vi "Get Node.vi"(8 "error in (no error)":errorcluster, 10 "Path in":string, 11 "Connection in":refnum<class "Connection.lvclass">) -> (0 "error out":errorcluster, 2 "Node out":refnum<class "TreeNode.lvclass">, 3 "Connection out":refnum<class "Connection.lvclass">)   [LabVIEW 2015, in "MDSplus.lvlib" / "Connection.lvclass"]
uses:
  <vilib>/MDSplus_LV2015/Classes/Connection_Class/Connection.lvclass
  <vilib>/MDSplus_LV2015/Classes/Data_Class/TreeNode_Class/TreeNode.lvclass
  <vilib>/MDSplus_LV2015/Classes/Connection_Class/Connection.lvclass/Connection.ctl
  <vilib>/MDSplus_LV2015/Classes/Data_Class/Data.lvclass
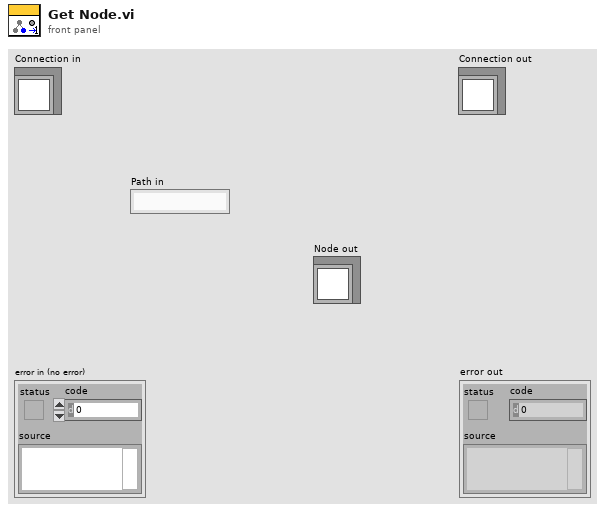
[diagram p1: front panel]
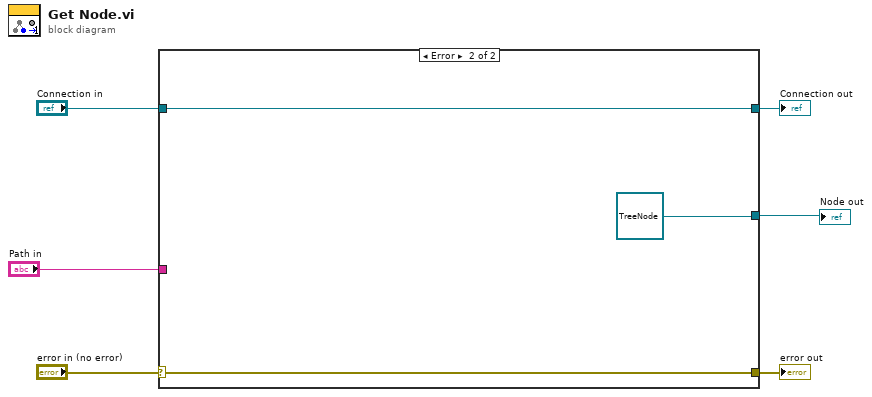
[diagram p0: block diagram]
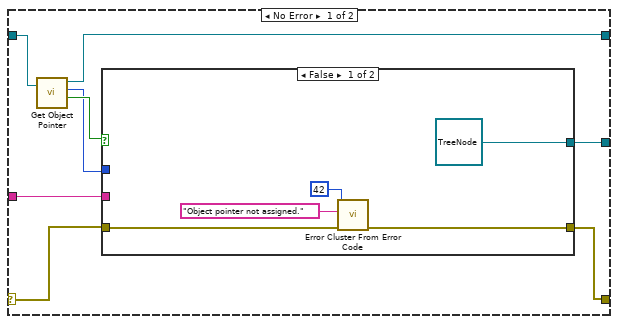
[diagram p2: hidden frame]
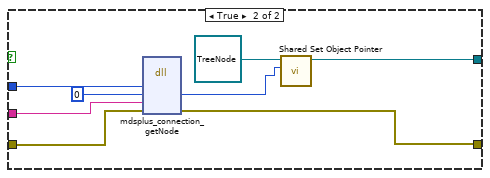
[diagram p3: hidden frame]
diagram:
  n1 = case shown="Error" "error in (no error)" {
    selector: "error in (no error)" -> [w10 w30]
    tunnel: [w9 w30] -> w5
    tunnel: [w13 w29] -> w3
    tunnel: "Connection in" -> [w14 w29]
    tunnel: "Path in" -> [w8 _]
    tunnel: [w7 refnum<class "TreeNode.lvclass"> refnum ("TreeNode")] -> w1
    frame No Error {
      n2 = call <vilib>:"Get Object Pointer.vi"("Connection in"=w14) -> ("Assigned object pointer?"=w12:bool, "Object Pointer"=w11:i64, "Connection out"=w13:refnum<class "Connection.lvclass">)  [unwired: 7 in, 1 out]
      n3 = case shown="False" w12 {
        tunnel: w11 -> [_ w26]
        tunnel: w10 -> [w17 w25]
        tunnel: [w16 w23] -> w9
        tunnel: w8 -> [_ w24]
        tunnel: [refnum<class "TreeNode.lvclass"> refnum ("TreeNode") w20] -> w7
        frame False {
          n4 = call <vilib>:"Error Cluster From Error Code.vi"("error in (no error)"=w17, "error message (\"\")"="Object pointer not assigned." ("error message (\"\")"), "error code (0)"=42) -> ("error out"=w16:errorcluster)  [unwired: 6 in]
        }
        frame True {
          n5 = dll-call lib="MDSobjectsLVShr" fn="mdsplus_connection_getNode"("lvConnectionPtr"=w26, "lvTreeNodePtrOut"=i64 0 ("lvDataPtrOut"), "PathIn"=w24, "error"=w25) -> ("lvTreeNodePtrOut"=w21:i64, "error"=w23:errorcluster)  [unwired: 6 in, 2 out]
          n6 = call <vilib>:"Shared Set Object Pointer.vi"("Object Pointer"=w21, "Data in"=refnum<class "TreeNode.lvclass"> refnum ("TreeNode")) -> ("Data out"=w20:refnum<class "TreeNode.lvclass">)  [unwired: 9 in]
        }
      }
    }
    frame Error {
    }
  }
  "error out" <- w5
  "Connection out" <- w3
  "Node out" <- w1
